vi "624 Fast Talon Read Sensor.vi"(9 "Reset?":bool, 11 "MotorControlDevRef":T1={"DeviceStatus"={"status"=FALSE, "code"=0, "source"=""}, "Type"=enum."PWM", "PWM"={"PWM Channel"=enum."Invalid", "DeadBand"={"Name"="", "maxPositivePwm"=0, "minPositivePwm"=0, "centerPwm"=0, "maxNegativePwm"=0, "minNegativePwm"=0, "angularRange"=0}}, "CAN"={"Device Number"=0, "Control Mode"=enum."Percent VBus", "Semaphore"=refnum, "Max Vout"=12.0, "TalonSRX Control Mode"=enum."Percent VBus"}, "Invert"=FALSE}) -> (0 "V Div By 4":bool, 1 "Current":dbl, 2 "Sensor Position":dbl, 3 "Sensor RPM":dbl)   [LabVIEW 2015]
uses:
  <vilib>/Rock Robotics/WPI/MotorControl/WPI_MotorControlDeviceRef.ctl
  <vilib>/Rock Robotics/WPI/MotorControl/WPI_MotorControlType.ctl
  <vilib>/Rock Robotics/SystemInterfaces/DIO/FPGA_DIOPWMChannel.ctl
  <vilib>/Rock Robotics/WPI/PWM/WPI_PWMDeadband.ctl
  <vilib>/Rock Robotics/WPI/CAN/Jaguar/SubVIs/WPI_CANJaguar_ControlMode.ctl
  <vilib>/Rock Robotics/WPI/CAN/TalonSRX/WPI_CANTalonSRX_APIControlMode.ctl
  <vilib>/Rock Robotics/WPI/CAN/TalonSRX/WPI_CANTalonSRX_MessageIDs.ctl
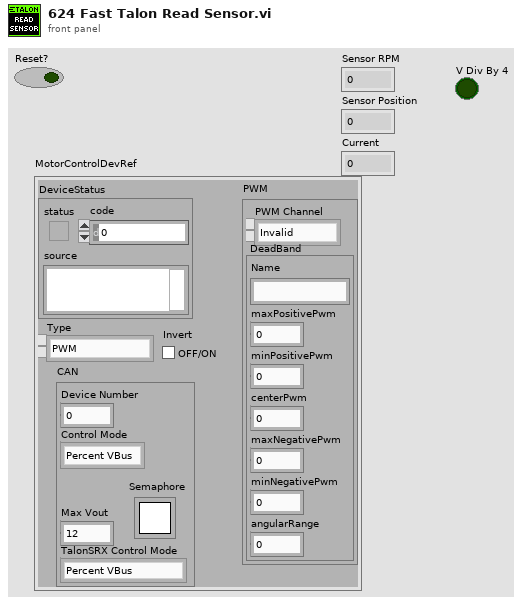
[diagram p1: front panel]
types:
  T1 = typedef "WPI_MotorControlDeviceRef.ctl" = cluster{"DeviceStatus":errorcluster, "Type":T2, "PWM":cluster{"PWM Channel":T3, "DeadBand":T4}, "CAN":cluster{"Device Number":u8, "Control Mode":T5, "Semaphore":T6, "Max Vout":dbl, "TalonSRX Control Mode":T7}, "Invert":bool}
  T2 = typedef "WPI_MotorControlType.ctl" = enum16{"PWM", "CAN", "CANTalonSRX"}
  T3 = typedef "FPGA_DIOPWMChannel.ctl" = enum8{"PWM 0", "PWM 1", "PWM 2", "PWM 3", "PWM 4", "PWM 5", "PWM 6", "PWM 7", "PWM 8", "PWM 9", "PWM MXP 0", "PWM MXP 1", "PWM MXP 2", "PWM MXP 3", "PWM MXP 4", "PWM MXP 5", "PWM MXP 6", "PWM MXP 7", "PWM MXP 8", "PWM MXP 9", "Invalid"}
  T4 = typedef "WPI_PWMDeadband.ctl" = cluster{"Name":string, "maxPositivePwm":i32, "minPositivePwm":i32, "centerPwm":i32, "maxNegativePwm":i32, "minNegativePwm":i32, "angularRange":u16}
  T5 = typedef "WPI_CANJaguar_ControlMode.ctl" = enum8{"Percent VBus", "Current", "Speed", "Position", "Voltage"}
  T6 = typedef "Semaphore RefNum" = refnum<k1>
  T7 = typedef "WPI_CANTalonSRX_APIControlMode.ctl" = enum8{"Percent VBus", "Speed", "Position", "Slave", "Unchanged / Invalid", "Voltage Compensation", "Current", "Motion Profile"}
  T8 = typedef "WPI_CANTalonSRX_MessageIDs.ctl" = u32
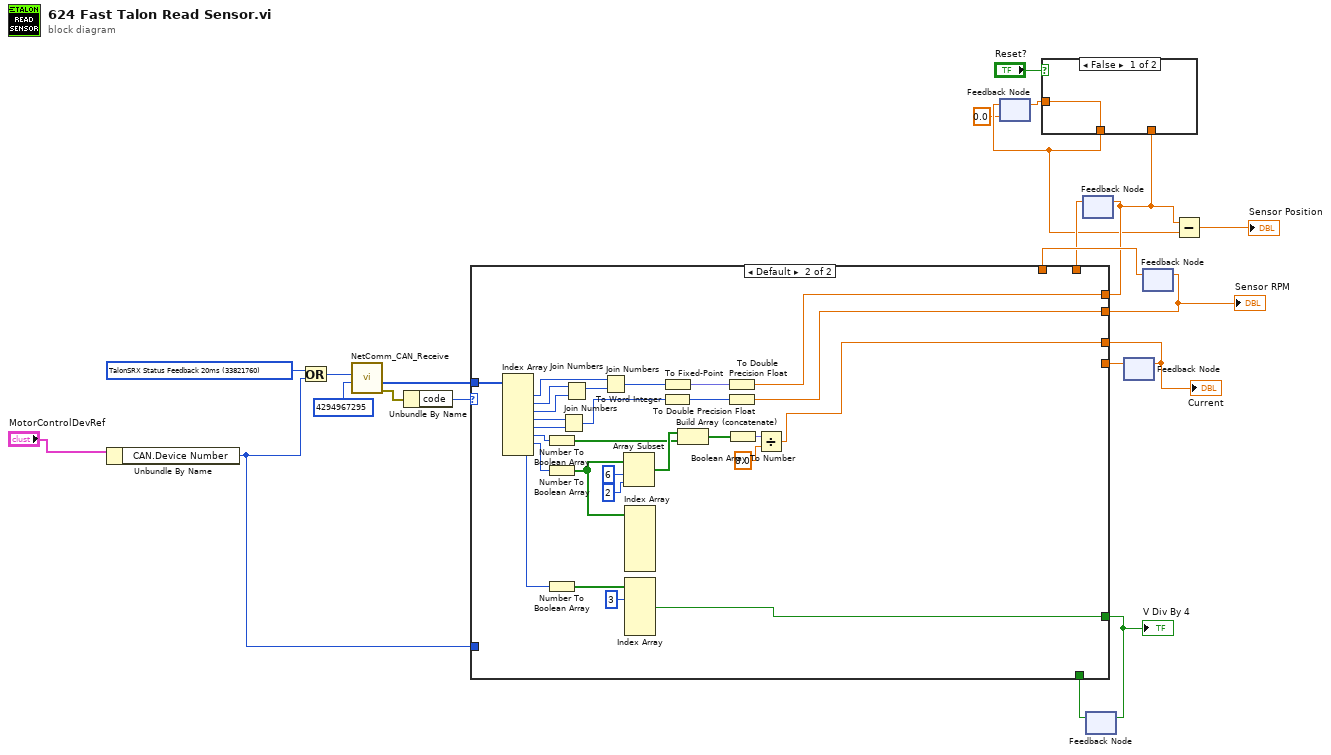
[diagram p0: block diagram]
diagram:
  w18 = T8 33821760 items=["TalonSRX Control General 10ms"=33816576, "TalonSRX Control Rates Slow"=33816640, "TalonSRX Control ClearFlags Slow"=33816704, "TalonSRX Status General 10ms"=33821696, "TalonSRX Status Feedback 20ms"=33821760, "TalonSRX Status Enc 100ms"=33821824, "TalonSRX Status AinTempVbat 100ms"=33821888, "TalonSRX Status Startup Once"=33821952, "TalonSRX Status Debug"=33822080, "TalonSRX Config SetGainsSlot0 A"=33823808, "TalonSRX Config SetGainsSlot0 B"=33823872, "TalonSRX Config SetGainsSlot1 A"=33823936, "TalonSRX Config SetGainsSlot1 B"=33824000, "TalonSRX Config SetSoftLimits"=33824064, "TalonSRX Config WebControl"=33824128, "TalonSRX Param Request"=33822720, "TalonSRX Param Response"=33822784, "TalonSRX Param Set"=33822848]
  n1 = Unbundle By Name("MotorControlDevRef") -> ("CAN.Device Number"=w8:u8)
  n2 = Or(x=w18, y=w8) -> (x .or. y?=w17:T8)
  n3 = call <vilib>:"NetComm_CAN_Receive.vi"("Message ID Mask"=u32 4294967295, "Message ID"=w17) -> ("error out"=w20:errorcluster, "Data"=w16:u8[])  [unwired: 6 in, 2 out]
  n4 = Unbundle By Name(w20) -> ("code"=w21:i32)
  n5 = feedback #1(0.0) -> (w4:dbl)
  n6 = feedback #2() -> (w9:dbl)  [unwired: 1 in]
  n7 = feedback #3() -> (w14:bool)  [unwired: 1 in]
  n8 = feedback #4() -> (w12:dbl)  [unwired: 1 in]
  n9 = feedback #5() -> (w10:dbl)  [unwired: 1 in]
  n10 = case shown="Default" w21 {
    tunnel: w8 -> [_ _]
    tunnel: w16 -> [_ w53]
    tunnel: [w22 w29] -> w5
    tunnel: [w23 w28] -> w11
    tunnel: [w24 w27] -> w13
    tunnel: [w25 w26] -> w15
    tunnel: w14 -> [w25 _]
    tunnel: w12 -> [w24 _]
    tunnel: w10 -> [w23 _]
    tunnel: w9 -> [w22 _]
    frame -44087 {
    }
    frame Default {
      n11 = Index Array(array=w53) -> (element #1=w45:u8, element #2=w47:u8, element #3=w44:u8, element #4=w43:u8, element #5=w42:u8, element #6=w40:u8, element #7=w39:u8, element #8=w36:u8)  [unwired: 8 in]
      n12 = Number To Boolean Array(number=w40) -> (Boolean array=w32:bool[])
      n13 = Number To Boolean Array(number=w39) -> (Boolean array=w52:bool[])
      n14 = Number To Boolean Array(number=w36) -> (Boolean array=w35:bool[])
      n15 = Join Numbers(hi=w43, lo=w42) -> ((hi.lo)=w41:u16)
      n16 = Join Numbers(hi=w47, lo=w44) -> ((hi.lo)=w46:u16)
      n17 = Join Numbers(hi=w45, lo=w46) -> ((hi.lo)=w31:u32)
      n18 = Array Subset(array=w52, index=6, length=2) -> (w33:bool[])
      n19 = Index Array(array=w52) -> ()  [unwired: 6 in, 6 out]
      n20 = Index Array(array=w35, index #1=3 ("index")) -> (element #2=w26:bool)  [unwired: 4 in, 4 out]
      n21 = To Word Integer(number=w41) -> (16bit integer=w34:i16)
      n22 = To Fixed-Point(number=w31) -> (fixed-point=w30:fxp<+/-,24,24>)  [unwired: 1 in]
      n23 = Build Array (concatenate)(w33, w32) -> (w50:bool[])
      n24 = To Double Precision Float(number=w30) -> (double precision float=w29:dbl)
      n25 = To Double Precision Float(number=w34) -> (double precision float=w28:dbl)
      n26 = Boolean Array To Number(Boolean array=w50) -> (number=w49:fxp<+/-,11,11>)
      n27 = Divide(x=w49, y=8.0) -> (x/y=w27:dbl)
    }
  }
  "Sensor RPM" <- w11
  "Current" <- w13
  "V Div By 4" <- w15
  n28 = case shown="False" "Reset?" {
    tunnel: [w54 w55] -> w6
    tunnel: w5 -> [_ w55]
    tunnel: w4 -> [w54 _]
    frame False {
    }
    frame True {
    }
  }
  n29 = feedback-in #1(w6) -> ()
  n30 = feedback-in #2(w5) -> ()
  n31 = feedback-in #3(w15) -> ()
  n32 = feedback-in #4(w13) -> ()
  n33 = feedback-in #5(w11) -> ()
  n34 = Subtract(x=w5, y=w4) -> (x-y=→"Sensor Position":dbl)
